vi "Sample Transfer Stop Freezers and Blowers.vi"(8 "error in (no error)":errorcluster, 11 "cRIO-CO2 in":refnum<class "cRIO-CO2.lvclass">) -> (0 "error out":errorcluster, 3 "cRIO-CO2 out":refnum<class "cRIO-CO2.lvclass">)   [LabVIEW 2015, in "cRIO-Carbondioxide.lvlib" / "cRIO-CO2.lvlib" / "cRIO-CO2.lvclass"]
uses:
  cRIO-CO2.lvclass
  cRIO-CO2.lvclass/cRIO-CO2.ctl
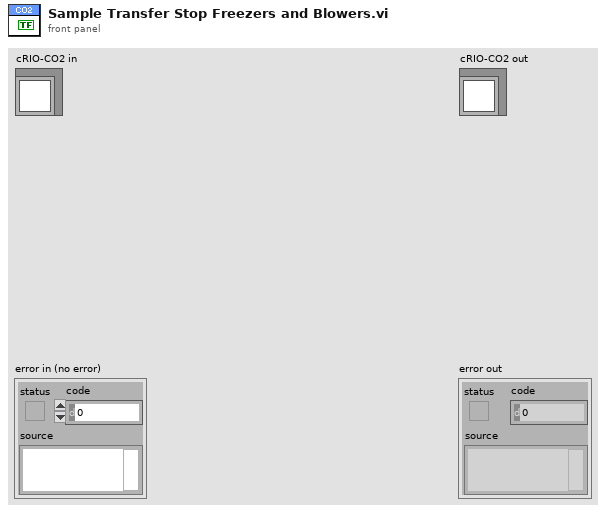
[diagram p1: front panel]
types:
  T1 = typedef "Sample Transfer Container Enumerator.ctl" = enum16{"None", "Sample 1", "Sample 2", "Sample 3", "Sample 4", "Sample 5", "Storage 01", "Storage 02", "Storage 03", "Storage 04", "Storage 05", "Storage 06", "Storage 07", "Storage 08", "Storage 09", "Storage 10", "Storage 11", "Storage 12", "Syringe", "Undefined"}
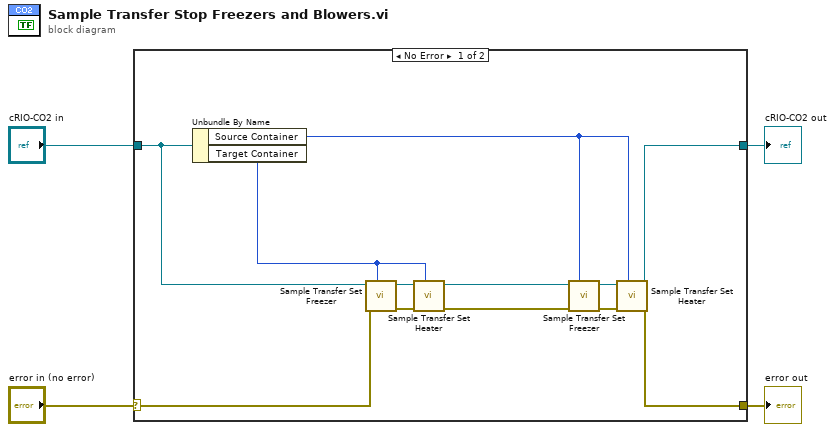
[diagram p0: block diagram]
diagram:
  n1 = case shown="No Error" "error in (no error)" {
    selector: "error in (no error)" -> [w15 w18]
    tunnel: [w9 w18] -> w3
    tunnel: [w8 w17] -> w1
    tunnel: "cRIO-CO2 in" -> [w16 w17]
    frame No Error {
      n2 = Unbundle By Name(w16) -> ("Source Container"=w11:T1, "Target Container"=w7:T1)
      n3 = call "Sample Transfer Set Freezer.vi"("Container"=w7, "error in (no error)"=w15, "cRIO-CO2 in"=w16) -> ("error out"=w6:errorcluster, "cRIO-CO2 out"=w5:refnum<class "cRIO-CO2.lvclass">)  [unwired: 6 in, 1 out]
      n4 = call "Sample Transfer Set Heater.vi"("Container"=w7, "error in (no error)"=w6, "cRIO-CO2 in"=w5) -> ("error out"=w13:errorcluster, "cRIO-CO2 out"=w12:refnum<class "cRIO-CO2.lvclass">)  [unwired: 6 in, 1 out]
      n5 = call "Sample Transfer Set Freezer.vi"("Container"=w11, "error in (no error)"=w13, "cRIO-CO2 in"=w12) -> ("error out"=w14:errorcluster, "cRIO-CO2 out"=w10:refnum<class "cRIO-CO2.lvclass">)  [unwired: 6 in, 1 out]
      n6 = call "Sample Transfer Set Heater.vi"("Container"=w11, "error in (no error)"=w14, "cRIO-CO2 in"=w10) -> ("error out"=w9:errorcluster, "cRIO-CO2 out"=w8:refnum<class "cRIO-CO2.lvclass">)  [unwired: 6 in, 1 out]
    }
    frame Error {
    }
  }
  "error out" <- w3
  "cRIO-CO2 out" <- w1
